vi "Read State Sample Message.vi"(8 "error in (no error)":errorcluster, 11 "State Sample Message in":refnum<class "State Sample Message.lvclass">) -> (0 "error out":errorcluster, 2 "State Sample":refnum<class "RDS State.lvclass">, 3 "State Sample Message out":refnum<class "State Sample Message.lvclass">)   [LabVIEW 2015, in "RDS Child Messages.lvlib" / "State Sample Message.lvclass"]
uses:
  State Sample Message.lvclass
  RDS State Tracker/RDS State/RDS State.lvclass
  State Sample Message.lvclass/State Sample Message.ctl
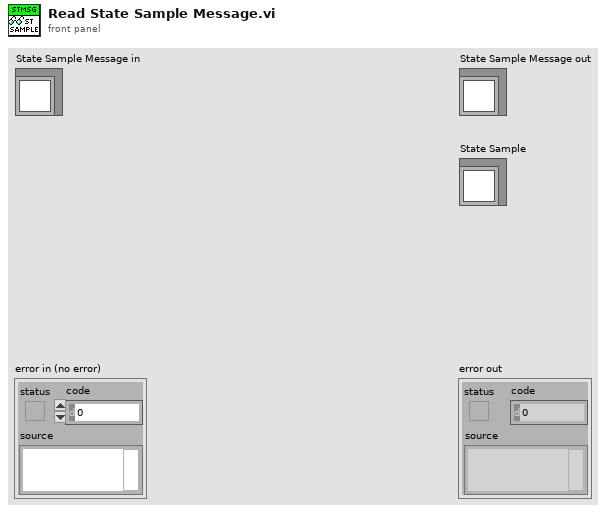
[diagram p1: front panel]
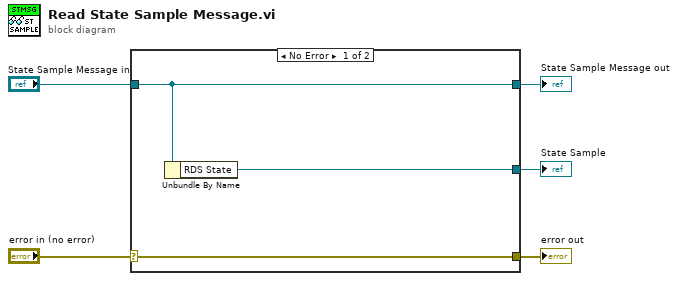
[diagram p0: block diagram]
diagram:
  n1 = case shown="No Error" "error in (no error)" {
    selector: "error in (no error)" -> [w8 w9]
    tunnel: [w8 w9] -> w4
    tunnel: [w7 w10] -> w2
    tunnel: "State Sample Message in" -> [w7 w10]
    tunnel: [w6 _] -> w1
    frame No Error {
      n2 = Unbundle By Name(w7) -> ("RDS State"=w6:refnum<class "RDS State.lvclass">)
    }
    frame Error {
    }
  }
  "error out" <- w4
  "State Sample Message out" <- w2
  "State Sample" <- w1
